vi "Init Instr In Vars.vi"(8 "error in (no error)":errorcluster, 10 "Chassis Present":bool[](array[boolean]), 11 "Acquisition Loop Data in":T1) -> (0 "error out":errorcluster, 3 "Acquisition Loop Data out":T1)   [LabVIEW 2018]
doc: "Pull input variable references for use during acquisition."
uses:
  Private Controls/Acquisition Loop Data.ctl
  RT - Instrument IO.lvlib
  FPGA/FPGA VI Reference.ctl
panel:
  out "appended array":errorcluster[](array[cluster])
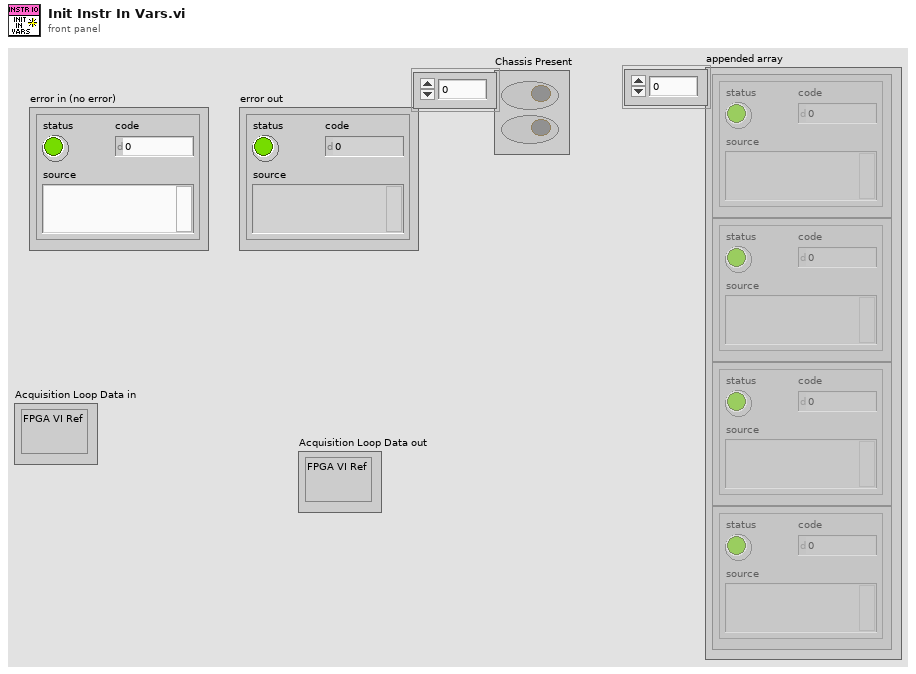
[diagram p1: front panel]
types:
  T1 = typedef "RT - Instrument IO.lvlib/Acquisition Loop Data.ctl" = cluster{"FPGA VI Ref":T2}
  T2 = typedef "FPGA VI Reference.ctl" = refnum<k20>
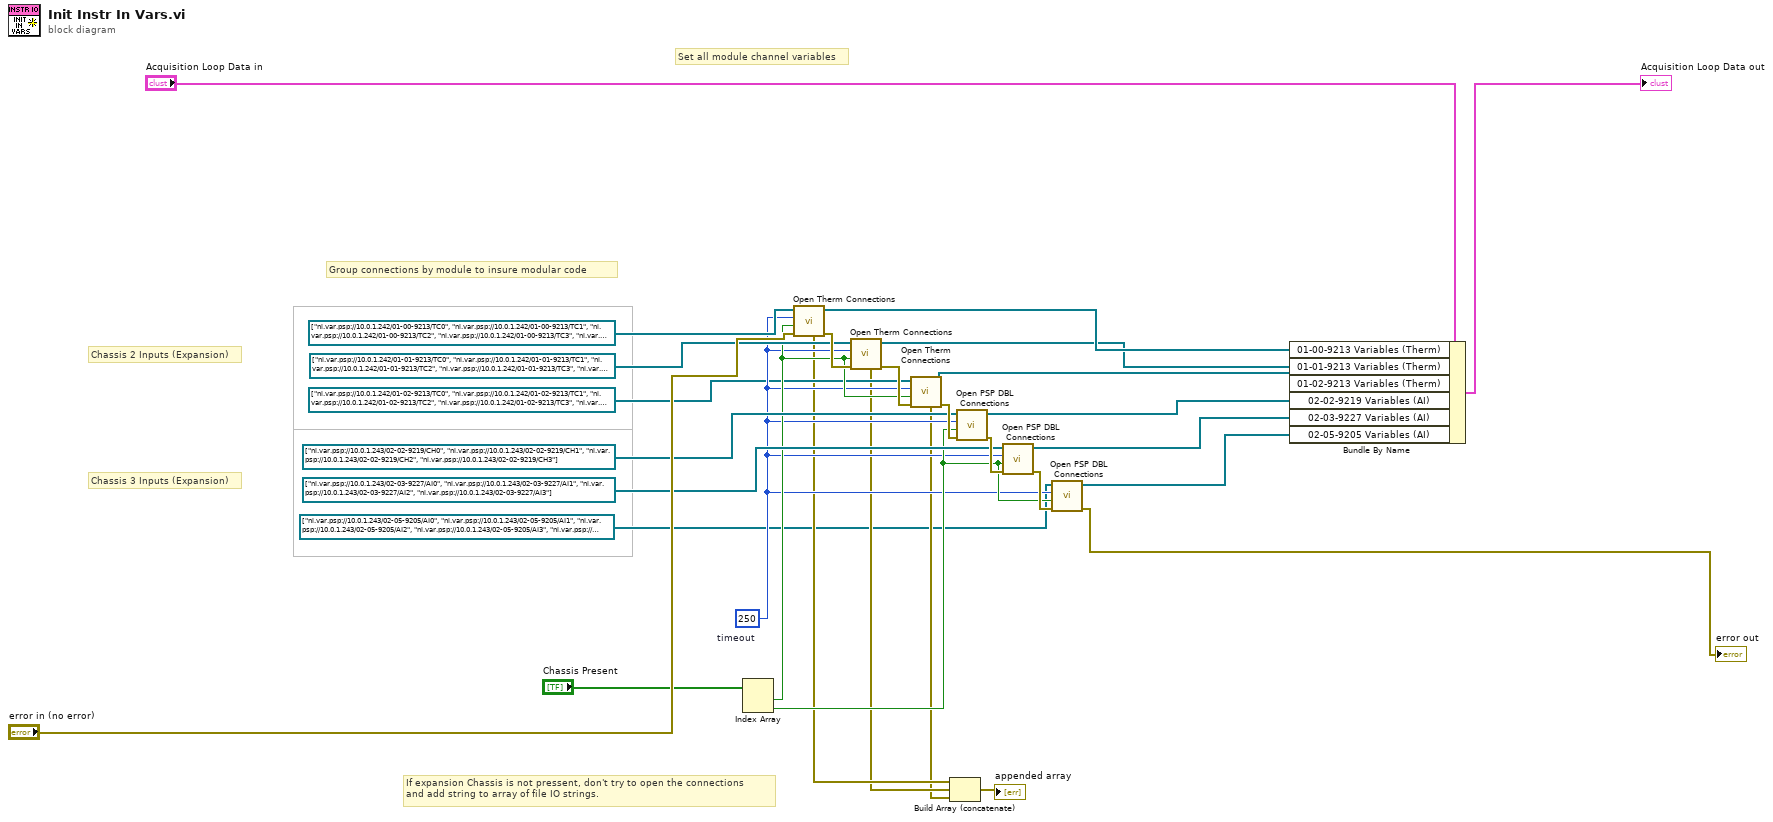
[diagram p0: block diagram]
diagram:
  w8 = 250  # timeout
  # "If expansion Chassis is not pressent, don't try to open the connections\nand add string to array of file IO strings."
  # "Group connections by module to insure modular code"
  # "Chassis 3 Inputs (Expansion)"
  # "Chassis 2 Inputs (Expansion)"
  # "Set all module channel variables"
  n1 = Index Array(array="Chassis Present") -> (element #1=w10:bool, element #2=w11:bool)  [unwired: 2 in]
  n2 = call "Open Therm Connections.vi"("error in (no error)"="error in (no error)", "Attempt Connection? (T)"=w10, "timeout (100ms)"=w8, "PSP Therm Channels in"=refnum<k21>[] ["ni.var.psp://10.0.1.242/01-00-9213/TC0", "ni.var.psp://10.0.1.242/01-00-9213/TC1", "ni.var.psp://10.0.1.242/01-00-9213/TC2", "ni.var.psp://10.0.1.242/01-00-9213/TC3", "ni.var.psp://10.0.1.242/01-00-9213/TC4", "ni.var.psp://10.0.1.242/01-00-9213/TC5", "ni.var.psp://10.0.1.242/01-00-9213/TC6", "ni.var.psp://10.0.1.242/01-00-9213/TC7", "ni.var.psp://10.0.1.242/01-00-9213/TC8", "ni.var.psp://10.0.1.242/01-00-9213/TC9", "ni.var.psp://10.0.1.242/01-00-9213/TC10", "ni.var.psp://10.0.1.242/01-00-9213/TC11", "ni.var.psp://10.0.1.242/01-00-9213/TC12", "ni.var.psp://10.0.1.242/01-00-9213/TC13", "ni.var.psp://10.0.1.242/01-00-9213/TC14", "ni.var.psp://10.0.1.242/01-00-9213/TC15"] ("01-00")) -> ("error out"=w26:errorcluster, "Opened Variables out"=w16:refnum<k21>[], "Errors"=w6:errorcluster[])  [unwired: 4 in, 1 out]
  n3 = call "Open Therm Connections.vi"("error in (no error)"=w26, "Attempt Connection? (T)"=w10, "timeout (100ms)"=w8, "PSP Therm Channels in"=refnum<k21>[] ["ni.var.psp://10.0.1.242/01-01-9213/TC0", "ni.var.psp://10.0.1.242/01-01-9213/TC1", "ni.var.psp://10.0.1.242/01-01-9213/TC2", "ni.var.psp://10.0.1.242/01-01-9213/TC3", "ni.var.psp://10.0.1.242/01-01-9213/TC4", "ni.var.psp://10.0.1.242/01-01-9213/TC5", "ni.var.psp://10.0.1.242/01-01-9213/TC6", "ni.var.psp://10.0.1.242/01-01-9213/TC7", "ni.var.psp://10.0.1.242/01-01-9213/TC8", "ni.var.psp://10.0.1.242/01-01-9213/TC9", "ni.var.psp://10.0.1.242/01-01-9213/TC10", "ni.var.psp://10.0.1.242/01-01-9213/TC11", "ni.var.psp://10.0.1.242/01-01-9213/TC12", "ni.var.psp://10.0.1.242/01-01-9213/TC13", "ni.var.psp://10.0.1.242/01-01-9213/TC14", "ni.var.psp://10.0.1.242/01-01-9213/TC15"] ("01-01")) -> ("error out"=w29:errorcluster, "Opened Variables out"=w15:refnum<k21>[], "Errors"=w5:errorcluster[])  [unwired: 4 in, 1 out]
  n4 = call "Open Therm Connections.vi"("error in (no error)"=w29, "Attempt Connection? (T)"=w10, "timeout (100ms)"=w8, "PSP Therm Channels in"=refnum<k21>[] ["ni.var.psp://10.0.1.242/01-02-9213/TC0", "ni.var.psp://10.0.1.242/01-02-9213/TC1", "ni.var.psp://10.0.1.242/01-02-9213/TC2", "ni.var.psp://10.0.1.242/01-02-9213/TC3", "ni.var.psp://10.0.1.242/01-02-9213/TC4", "ni.var.psp://10.0.1.242/01-02-9213/TC5", "ni.var.psp://10.0.1.242/01-02-9213/TC6", "ni.var.psp://10.0.1.242/01-02-9213/TC7", "ni.var.psp://10.0.1.242/01-02-9213/TC8", "ni.var.psp://10.0.1.242/01-02-9213/TC9", "ni.var.psp://10.0.1.242/01-02-9213/TC10", "ni.var.psp://10.0.1.242/01-02-9213/TC11", "ni.var.psp://10.0.1.242/01-02-9213/TC12", "ni.var.psp://10.0.1.242/01-02-9213/TC13", "ni.var.psp://10.0.1.242/01-02-9213/TC14", "ni.var.psp://10.0.1.242/01-02-9213/TC15"] ("01-02")) -> ("error out"=w25:errorcluster, "Opened Variables out"=w14:refnum<k21>[], "Errors"=w4:errorcluster[])  [unwired: 4 in, 1 out]
  n5 = Build Array (concatenate)(w6, w5, w4) -> (→"appended array":errorcluster[])
  n6 = call "Open PSP DBL Connections.vi"("error in (no error)"=w25, "Attempt Connection? (T)"=w11, "timeout (100ms)"=w8, "PSP Variables in"=refnum<k21>[] ["ni.var.psp://10.0.1.243/02-02-9219/CH0", "ni.var.psp://10.0.1.243/02-02-9219/CH1", "ni.var.psp://10.0.1.243/02-02-9219/CH2", "ni.var.psp://10.0.1.243/02-02-9219/CH3"] ("02-02")) -> ("error out"=w28:errorcluster, "Open Variables out"=w13:refnum<k21>[])  [unwired: 4 in, 2 out]
  n7 = call "Open PSP DBL Connections.vi"("error in (no error)"=w28, "Attempt Connection? (T)"=w11, "timeout (100ms)"=w8, "PSP Variables in"=refnum<k21>[] ["ni.var.psp://10.0.1.243/02-03-9227/AI0", "ni.var.psp://10.0.1.243/02-03-9227/AI1", "ni.var.psp://10.0.1.243/02-03-9227/AI2", "ni.var.psp://10.0.1.243/02-03-9227/AI3"] ("02-03")) -> ("error out"=w27:errorcluster, "Open Variables out"=w12:refnum<k21>[])  [unwired: 4 in, 2 out]
  n8 = call "Open PSP DBL Connections.vi"("error in (no error)"=w27, "Attempt Connection? (T)"=w11, "timeout (100ms)"=w8, "PSP Variables in"=refnum<k21>[] ["ni.var.psp://10.0.1.243/02-05-9205/AI0", "ni.var.psp://10.0.1.243/02-05-9205/AI1", "ni.var.psp://10.0.1.243/02-05-9205/AI2", "ni.var.psp://10.0.1.243/02-05-9205/AI3", "ni.var.psp://10.0.1.243/02-05-9205/AI4", "ni.var.psp://10.0.1.243/02-05-9205/AI5", "ni.var.psp://10.0.1.243/02-05-9205/AI6", "ni.var.psp://10.0.1.243/02-05-9205/AI7", "ni.var.psp://10.0.1.243/02-05-9205/AI16", "ni.var.psp://10.0.1.243/02-05-9205/AI17", "ni.var.psp://10.0.1.243/02-05-9205/AI18", "ni.var.psp://10.0.1.243/02-05-9205/AI19", "ni.var.psp://10.0.1.243/02-05-9205/AI20", "ni.var.psp://10.0.1.243/02-05-9205/AI21", "ni.var.psp://10.0.1.243/02-05-9205/AI22", "ni.var.psp://10.0.1.243/02-05-9205/AI23"] ("02-05")) -> ("error out"=→"error out":errorcluster, "Open Variables out"=w24:refnum<k21>[])  [unwired: 4 in, 2 out]
  n9 = Bundle By Name(cluster="Acquisition Loop Data in", "01-00-9213 Variables (Therm)"=w16, "01-01-9213 Variables (Therm)"=w15, "01-02-9213 Variables (Therm)"=w14, "02-02-9219 Variables (AI)"=w13, "02-03-9227 Variables (AI)"=w12, "02-05-9205 Variables (AI)"=w24) -> (→"Acquisition Loop Data out":T1)
